vi "bin_header_write.vi"(0 "New_BIN_FILE":path=path "/home/ageevvb/labview/EDF_READ/test.bin", 1 "CH_NUM":u8=4, 2 "Length":u16, 3 "Freq_d":u16=1000, 4 "Meta":string) -> (5 "refnum_out":refnum<file>)   [LabVIEW 2013]
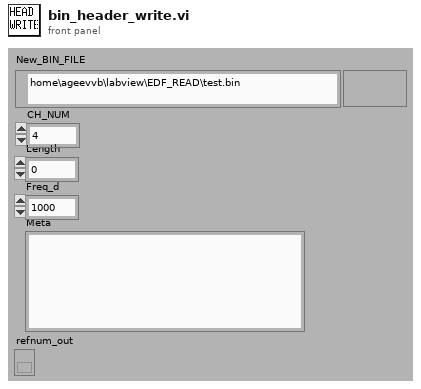
[diagram p1: front panel]
types:
  T1 = enum16{"open", "replace", "create", "open or create", "replace or create", "replace or create with confirmation"}
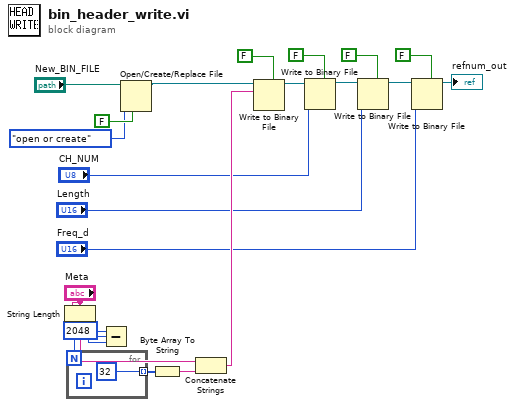
[diagram p0: block diagram]
diagram:
  n1 = String Length(string="Meta") -> (length=w20:i32)
  n2 = Subtract(x=2048, y=w20) -> (x-y=w18:i32)
  n3 = for {
    N: w18 -> [_]
    tunnel: [u8 32] -> w17 mode=indexing
  }
  n4 = Open/Create/Replace File(file path (use dialog)="New_BIN_FILE", operation (0:open)=T1."open or create", disable buffering (F)=FALSE ("advisory dialog? (display:T)")) -> (refnum out=w21:refnum<file>)  [unwired: 3 in, 2 out]
  n5 = Byte Array To String(unsigned byte array=w17) -> (string=w16:string)
  n6 = Concatenate Strings("Meta", w16) -> (w14:string)
  n7 = Write to Binary File(file (use dialog)=w21, data=w14, 5:FALSE ("prepend array or string size? (T)")) -> (refnum out=w13:refnum<file>)  [unwired: 3 in, 2 out]
  n8 = Write to Binary File(file (use dialog)=w13, data="CH_NUM", 5:FALSE ("prepend array or string size? (T)")) -> (refnum out=w12:refnum<file>)  [unwired: 3 in, 2 out]
  n9 = Write to Binary File(file (use dialog)=w12, data="Length", 5:FALSE ("prepend array or string size? (T)")) -> (refnum out=w11:refnum<file>)  [unwired: 3 in, 2 out]
  n10 = Write to Binary File(file (use dialog)=w11, data="Freq_d", 5:FALSE ("prepend array or string size? (T)")) -> (refnum out=→"refnum_out":refnum<file>)  [unwired: 3 in, 2 out]
